vi "ElapsedTimeToTimeStampedMessage.vi"(10 "Time Opened":timestamp, 11 "ElapsedTimeMessage":T2) -> (3 "TimeStampedMessage":T1)   [LabVIEW 2011, in "NetworkStreamReader.lvclass"]
doc: "Converts a messge with an elapsed time since the last reconnection between the writer and its corresponding reader endpoint to a message with a time stamp.\n\nJared Kirschner, 2012."
uses:
  NetworkStreamReader.lvclass
  Shared/ElapsedTimeMessage.ctl
  Shared/TimeStampedMessage.ctl
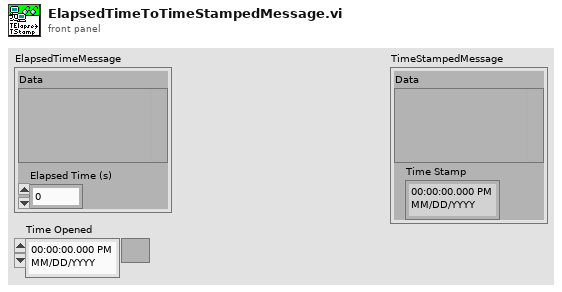
[diagram p1: front panel]
types:
  T1 = typedef "TimeStampedMessage.ctl" = cluster{"Data":variant, "Time Stamp":timestamp}
  T2 = typedef "ElapsedTimeMessage.ctl" = cluster{"Data":variant, "Elapsed Time (s)":dbl}
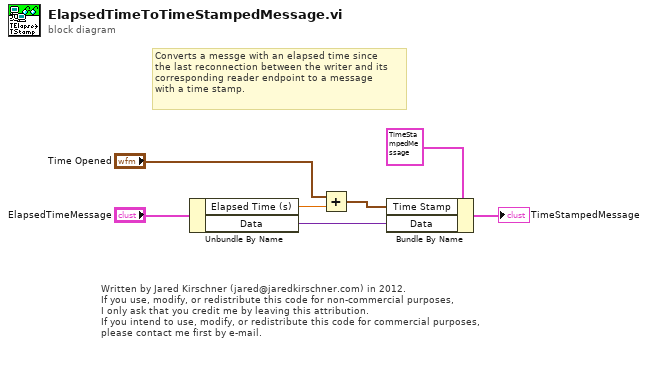
[diagram p0: block diagram]
diagram:
  # "Converts a messge with an elapsed time since\nthe last reconnection between the writer and its\ncorresponding reader endpoint to a message\nwith a time stamp."
  # "Written by Jared Kirschner (jared@jaredkirschner.com) in 2012.\nIf you use, modify, or redistribute this code for non-commercial purposes,\nI only ask that you credit me by leaving this attribution.\nIf you intend to use, modify, or redistribute this code for commercial purposes,\nplease contact me first by e-mail."
  n1 = Unbundle By Name("ElapsedTimeMessage") -> ("Elapsed Time (s)"=w5:dbl, "Data"=w6:variant)
  n2 = Add(x="Time Opened", y=w5) -> (x+y=w2:timestamp)
  n3 = Bundle By Name(cluster=T1 {"Data"=variant, "Time Stamp"=timestamp(0 s since 1904-01-01)} ("Message"), "Time Stamp"=w2, "Data"=w6) -> (→"TimeStampedMessage":T1)
